vi "Arrange VIWin - Arrange FP Controls Columns.vi"(0 "sorted controls":refnum<vi>[](array[refnum]), 1 "FP objects arrangement info":T1, 5 "sorted terminal boundaries":T2[](array[typedef]), 11 "error in":errorcluster) -> (15 "error out":errorcluster)   [LabVIEW 2015, in "Arrange VI Window.lvlib"]
uses:
  Arrange VI Window.lvlib
  <vilib>/Utility/miscctls.llb/LVRectTypeDef.ctl
  Arrange VIWin - FP Objects Arrangement Info.ctl
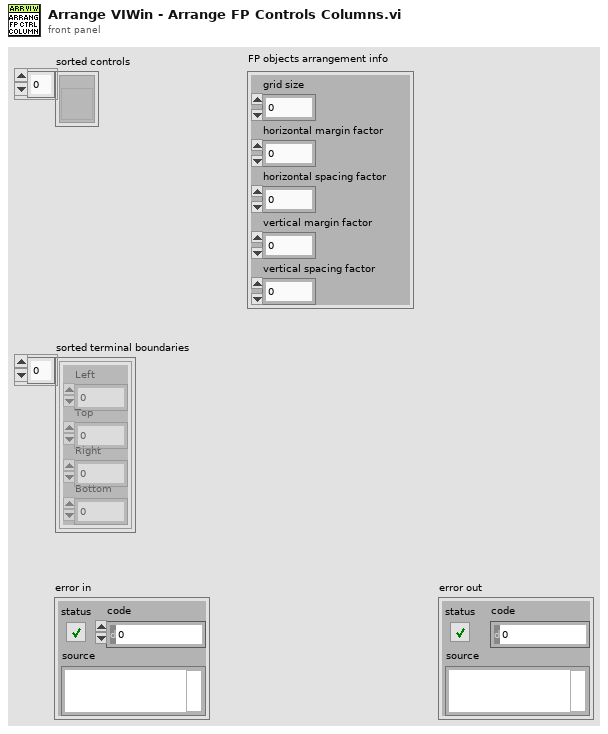
[diagram p1: front panel]
types:
  T1 = typedef "Arrange VI Window.lvlib/Arrange VIWin - FP Objects Arrangement Info.ctl" = cluster{"grid size":i32, "horizontal margin factor":i32, "horizontal spacing factor":i32, "vertical margin factor":i32, "vertical spacing factor":i32}
  T2 = typedef "LVRectTypeDef.ctl" = cluster{"Left":i16, "Top":i16, "Right":i16, "Bottom":i16}
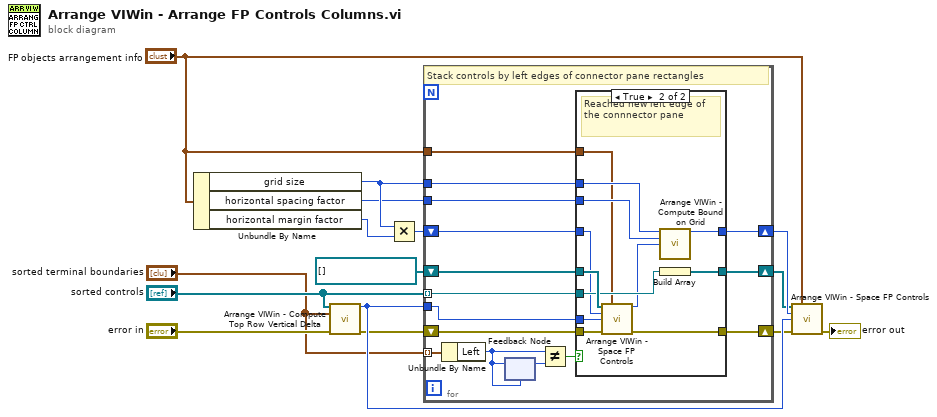
[diagram p0: block diagram]
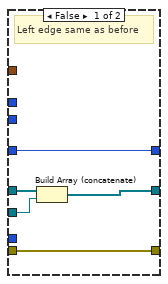
[diagram p2: hidden frame]
diagram:
  n1 = Unbundle By Name("FP objects arrangement info") -> ("grid size"=w14:i32, "horizontal spacing factor"=w2:i32, "horizontal margin factor"=w8:i32)
  n2 = call "Arrange VIWin - Compute Top Row Vertical Delta.vi"("controls"="sorted controls", "TermBnds[]"="sorted terminal boundaries", "error in"="error in") -> ("max vertical rectangle delta for controls from the top row"=w12:i16, "error out"=w9:errorcluster)  [unwired: 11 in]
  n3 = Multiply(x=w14, y=w8) -> (x*y=w7:i32)
  n4 = for {
    shift-right: [w29] -> w4
    shift-left: refnum<vi>[] [] -> [w28]
    shift-right: [w26] -> w13
    shift-left: w7 -> [w17]
    tunnel: "sorted controls" -> [w24] mode=indexing
    shift-right: [w18] -> w5
    shift-left: w9 -> [w25]
    tunnel: "sorted terminal boundaries" -> [w23] mode=indexing
    tunnel: w2 -> [w21]
    tunnel: w14 -> [w20]
    tunnel: w12 -> [w19]
    tunnel: "FP objects arrangement info" -> [w16]
    # "Stack controls by left edges of connector pane rectangles"
    n5 = Unbundle By Name(w23) -> ("Left"=w22:i16)
    n6 = feedback-in #1(w22) -> ()
    n7 = feedback #1(w22) -> (w30:i16)
    n8 = Not Equal?(x=w22, y=w30) -> (x != y?=w27:bool)
    n9 = case shown="True" w27 {
      tunnel: [w35 w47] -> w29
      tunnel: w28 -> [w34 w44]
      tunnel: [w33 w37] -> w26
      tunnel: w17 -> [w33 w41]
      tunnel: [w32 w46] -> w18
      tunnel: w25 -> [w32 w45]
      tunnel: w24 -> [w31 w43]
      tunnel: w21 -> [_ w38]
      tunnel: w20 -> [_ w39]
      tunnel: w19 -> [_ w42]
      tunnel: w16 -> [_ w36]
      frame False {
        # "Left edge same as before"
        n10 = Build Array (concatenate)(w34, w31) -> (w35:refnum<vi>[])
      }
      frame True {
        # "Reached new left edge of the connnector pane"
        n11 = call "Arrange VIWin - Space FP Controls.vi"("controls"=w44, "FP objects arrangement info"=w36, "left bound"=w41, "max vertical rectangle delta for controls from the top row"=w42, "error in"=w45) -> ("Max right location"=w40:i32, "error out"=w46:errorcluster)  [unwired: 9 in]
        n12 = call "Arrange VIWin - Compute Bound on Grid.vi"("grid size"=w39, "grid factor"=w38, "max location (not counting spacing and grid)"=w40) -> ("computed bound on the grid"=w37:i32)  [unwired: 12 in]
        n13 = Build Array(w43) -> (w47:refnum<vi>[])
      }
    }
  }
  n14 = call "Arrange VIWin - Space FP Controls.vi"("controls"=w4, "FP objects arrangement info"="FP objects arrangement info", "left bound"=w13, "max vertical rectangle delta for controls from the top row"=w12, "error in"=w5) -> ("error out"=→"error out":errorcluster)  [unwired: 9 in, 1 out]
